vi "LoadFromIni.vi"(8 "error in (no error)":errorcluster, 10 "Path":path, 11 "FTPConfig in":refnum<class "FTPConfig.lvclass">) -> (0 "error out":errorcluster, 3 "FTPConfig out":refnum<class "FTPConfig.lvclass">)   [LabVIEW 2020, in "FileSync -- FTP.lvlib" / "FTPConfig.lvclass"]
uses:
  FTPConfig.lvclass
  Def-FTP Server Info.vi
  FTPConfig.lvclass/FTPConfig.ctl
  <vilib>/Utility/config.llb/NI_LVConfig.lvlib
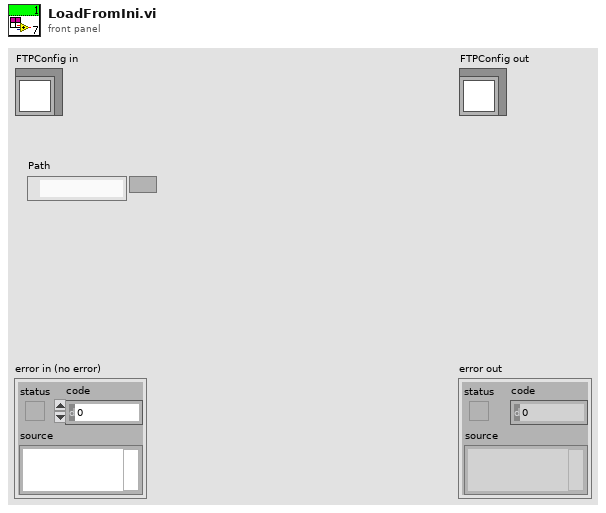
[diagram p1: front panel]
types:
  T1 = typedef "FileSync -- FTP.lvlib/FTPConfig.lvclass/Def-FTP Server Info.vi" = cluster{"address":string, "remote port":u16, "userName":string, "passWord":string, "RootDir":string}
  T2 = typedef "NI_LVConfig.lvlib/Config Data RefNum.ctl" = refnum<k1>
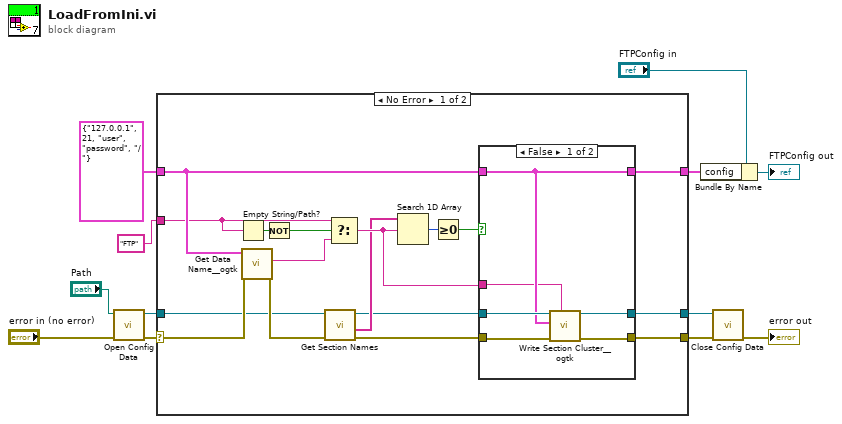
[diagram p0: block diagram]
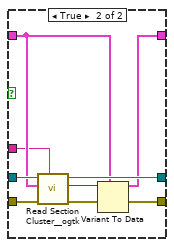
[diagram p2: hidden frame]
diagram:
  n1 = call <vilib>:"Open Config Data.vi"("error in (no error)"="error in (no error)", "configuration file path"="Path") -> ("error out"=w10:errorcluster, "refnum"=w11:T2)  [unwired: 7 in, 1 out]
  n2 = case shown="No Error" w10 {
    selector: w10 -> [w27 w45]
    tunnel: T1 {"address"="127.0.0.1", "remote port"=21, "userName"="user", "passWord"="password", "RootDir"="/"} -> [w26 w47]
    tunnel: "FTP" ("section") -> [w24 _]
    tunnel: w11 -> [w16 w46]
    tunnel: [w15 w45] -> w7
    tunnel: [w14 w46] -> w8
    tunnel: [w13 w47] -> w1
    frame No Error {
      n3 = Empty String/Path?(string/path=w24) -> (empty?=w22:bool)
      n4 = call <userlib>:"Get Data Name__ogtk.vi"("error in (no error)"=w27, "Data"=w26) -> ("error out"=w28:errorcluster, "Data Name"=w25:string)  [unwired: 7 in, 1 out]
      n5 = Not(x=w22) -> (.not. x?=w23:bool)
      n6 = call <vilib>:"Get Section Names.vi"("error in (no error)"=w28, "refnum"=w16) -> ("error out"=w18:errorcluster, "section names"=w19:string[], "refnum out"=w17:T2)  [unwired: 7 in]
      n7 = Select(t=w24, s=w23, f=w25) -> (s? t:f=w29:string)
      n8 = Search 1D Array(1D array=w19, element=w29) -> (index of element=w20:i32)  [unwired: 1 in]
      n9 = Greater Or Equal To 0?(x=w20) -> (x >= 0?=w21:bool)
      n10 = case shown="False" w21 {
        tunnel: w17 -> [w35 w44]
        tunnel: [w34 w43] -> w14
        tunnel: w18 -> [w32 w42]
        tunnel: [w33 w40] -> w15
        tunnel: w26 -> [w31 w38]
        tunnel: [w31 w39] -> w13
        tunnel: w29 -> [w30 w37]
        frame False {
          n11 = call <userlib>:"Write Section Cluster__ogtk.vi"("section (optional)"=w30, "error in (no error)"=w32, "Section Formatted Cluster"=w31, "refnum"=w35) -> ("error out"=w33:errorcluster, "dup refnum"=w34:T2)  [unwired: 6 in]
        }
        frame True {
          n12 = call <userlib>:"Read Section Cluster__ogtk.vi"("section (optional)"=w37, "error in (no error)"=w42, "Section Formatted Cluster Type"=w38, "refnum"=w44) -> ("error out"=w41:errorcluster, "Section Formatted Cluster"=w36:variant, "dup refnum"=w43:T2)  [unwired: 3 in, 2 out]
          n13 = Variant To Data(error in=w41, type=w38, Variant=w36) -> (data=w39:T1, error out=w40:errorcluster)
        }
      }
    }
    frame Error {
    }
  }
  n14 = Bundle By Name(cluster="FTPConfig in", "config"=w1) -> (→"FTPConfig out":refnum<class "FTPConfig.lvclass">)
  n15 = call <vilib>:"Close Config Data.vi"("error in (no error)"=w7, "refnum"=w8) -> ("error out"=→"error out":errorcluster)  [unwired: 8 in, 1 out]
